vi "Get RPM.vi"(8 "error in (no error)":errorcluster, 9 "Simulation Mode":string, 10 "Acquisition Metrics in":T1={"Total_Samples"=0, "rpm"=1000.0}, 11 "task/channels in":refnum<k21>) -> (0 "error out":errorcluster, 3 "Acquisition Metrics out":T1={"Total_Samples"=0, "rpm"=1000.0})   [LabVIEW 2026, in "Acquisition.lvlib"]
uses:
  Acquisition.lvlib
  Controls/Acquisition Metrics.ctl
  <vilib>/DAQmx/read.llb/DAQmx Read (Counter DBL 1Chan 1Samp).vi
  <vilib>/DAQmx/miscellaneous.llb/DAQmx Fill In Error Info.vi
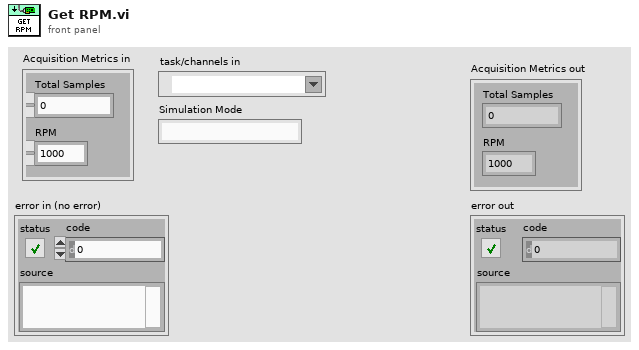
[diagram p1: front panel]
types:
  T1 = typedef "Acquisition.lvlib/Acquisition Metrics.ctl" = cluster{"Total_Samples":i64, "rpm":dbl}
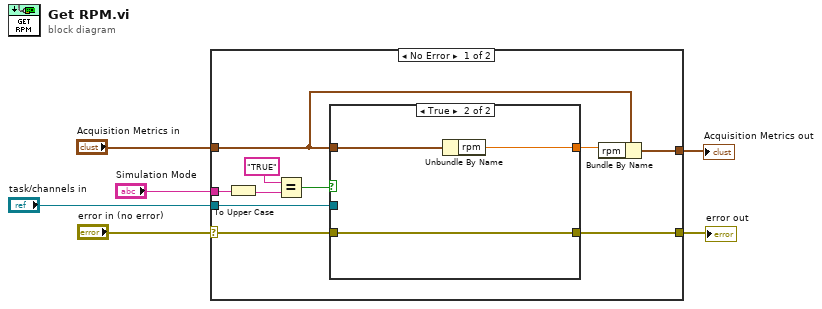
[diagram p0: block diagram]
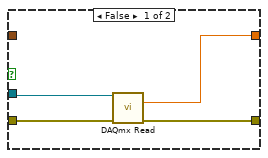
[diagram p2: hidden frame]
diagram:
  n1 = case shown="No Error" "error in (no error)" {
    selector: "error in (no error)" -> [w14 w25]
    tunnel: "Acquisition Metrics in" -> [w11 w24]
    tunnel: [w13 w25] -> w4
    tunnel: "Simulation Mode" -> [w16 _]
    tunnel: [w10 w24] -> w2
    tunnel: "task/channels in" -> [w9 _]
    frame No Error {
      n2 = To Upper Case(1:w16) -> (0:w8:string)
      n3 = Equal?(x="TRUE" ("y"), y=w8) -> (x = y?=w15:bool)
      n4 = case shown="True" w15 {
        tunnel: [w18 w23] -> w12
        tunnel: w11 -> [_ w22]
        tunnel: w14 -> [w20 w21]
        tunnel: [w19 w21] -> w13
        tunnel: w9 -> [w17 _]
        frame False {
          n5 = call-poly <vilib>:"DAQmx Read.vi"("task/channels in"=w17, "error in"=w20) -> ("data"=w18:dbl, "error out"=w19:errorcluster)  [unwired: 11 in, 1 out]
        }
        frame True {
          n6 = Unbundle By Name(w22) -> ("rpm"=w23:dbl)
        }
      }
      n7 = Bundle By Name(cluster=w11, "rpm"=w12) -> (w10:T1)
    }
    frame Error {
    }
  }
  "error out" <- w4
  "Acquisition Metrics out" <- w2
